vi "ActuatorCal.vi"() -> ()   [LabVIEW 2017]
panel:
  out "Saving Data":bool
  out "Filename In":path caption="Filename Out"
  in  "Stop To Calc Stats":bool
  out "Filename Out":path
  in  "Write to .lvm":bool
  in  "stop (F)":bool
  out "Total Samples":dbl
  out "Minimum":dbl
  out "Maximum":dbl
  out "Standard Dev":dbl
  out "RMS":dbl
  out "Arithmetic Mean":dbl
  out "Raw":dbl
  out "Waveform Chart":dynamicdata(graph)
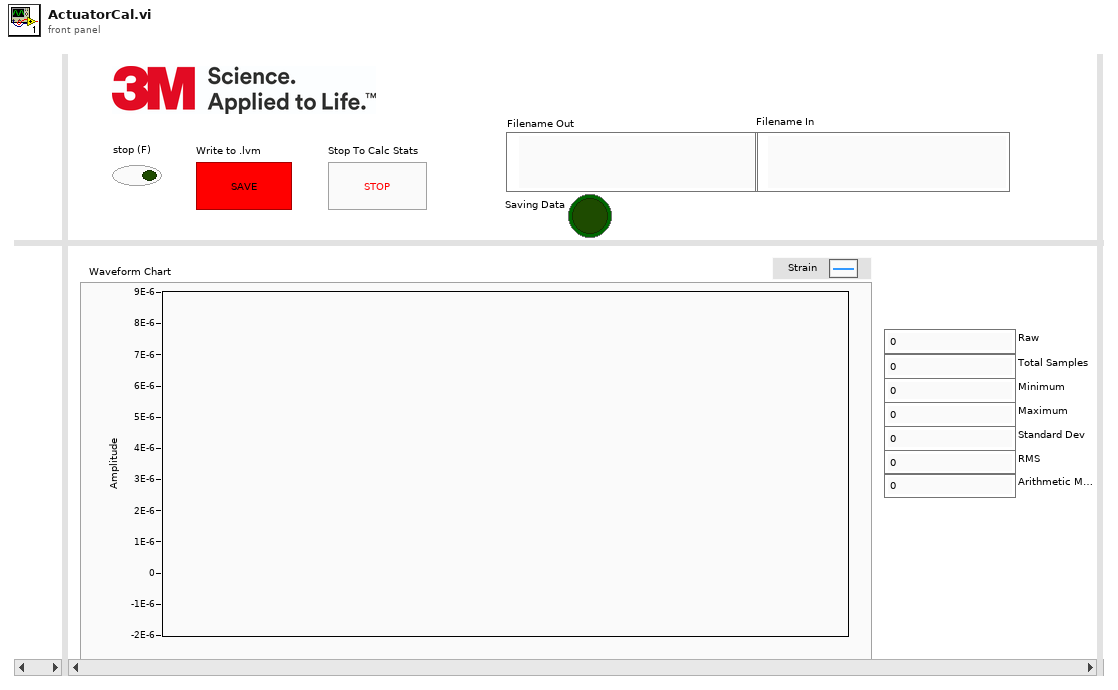
[diagram p1: front panel]
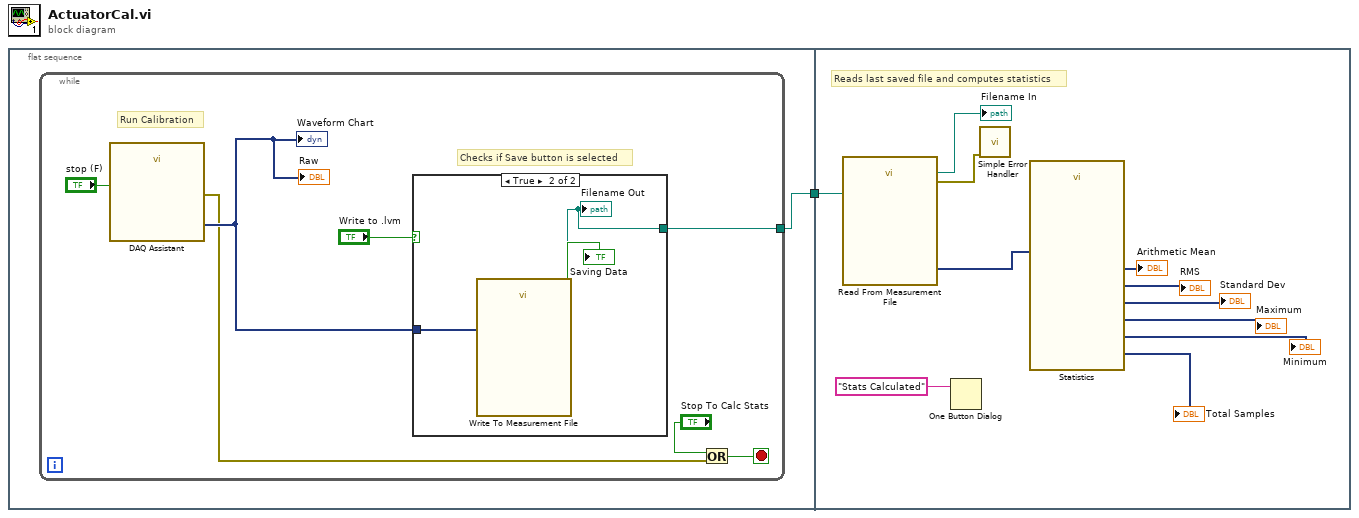
[diagram p0: block diagram]
diagram:
  n1 = flat-sequence {
    tunnel: [w2] -> w1
    tunnel: w1 -> [w22]
    frame #0 {
      n2 = while {
        tunnel: [w6] -> w2
        stop <- w3 stop-if-true
        # "Run Calibration"
        # "Checks if Save button is selected"
        n3 = call "DAQ Assistant"("stop (F)"="stop (F)") -> ("data"=w7:dynamicdata, "error out"=w5:errorcluster)  [unwired: 15 in, 2 out]
        "Waveform Chart" <- w7
        "Raw" <- w7
        n4 = case shown="True" "Write to .lvm" {
          tunnel: w7 -> [_ w12]
          tunnel: [_ w10] -> w6
          frame False {
          }
          frame True {
            n5 = call "Write To Measurement File"("Signals"=w12) -> ("Filename Out"=w10:path, "Saving Data"=→"Saving Data":bool)  [unwired: 16 in, 1 out]
            "Filename Out" <- w10
          }
        }
        n6 = Or(x="Stop To Calc Stats", y=w5) -> (x .or. y?=w3:bool)
      }
    }
    frame #1 {
      # "Reads last saved file and computes statistics"
      n7 = call "Read From Measurement File"("Filename"=w22) -> ("error out"=w13:errorcluster, "Filename Out"=→"Filename In":path, "Signals"=w23:dynamicdata)  [unwired: 5 in, 3 out]
      n8 = One Button Dialog(message="Stats Calculated") -> ()  [unwired: 1 in, 1 out]
      n9 = call <vilib>:"Simple Error Handler.vi"("error in (no error)"=w13) -> ()  [unwired: 4 in, 5 out]
      n10 = call "Statistics"("Signals"=w23) -> ("Total Samples"=→"Total Samples":dynamicdata, "Standard Dev"=→"Standard Dev":dynamicdata, "RMS"=→"RMS":dynamicdata, "Arithmetic Mean"=→"Arithmetic Mean":dynamicdata, "Minimum"=→"Minimum":dynamicdata, "Maximum"=→"Maximum":dynamicdata)  [unwired: 20 in, 1 out]
    }
  }
